vi "GetClickSelection.vi"(1 "Boundaries":cluster{"low":i32, "high":i32}[](array[cluster])=[{"low"=10, "high"=22}, {"low"=30, "high"=42}, {"low"=50, "high"=62}], 2 "Mouse":T1) -> (0 "selection":i32)   [LabVIEW 2012]
uses:
  <vilib>/Utility/miscctls.llb/LVMouseTypeDef.ctl
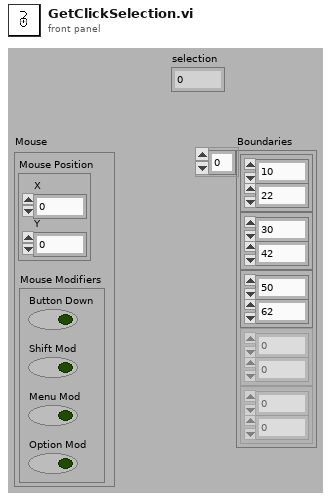
[diagram p1: front panel]
types:
  T1 = typedef "LVMouseTypeDef.ctl" = cluster{"Mouse Position":cluster{"X":i32, "Y":i32}, "Mouse Modifiers":cluster{"Button Down":bool, "Shift Mod":bool, "Menu Mod":bool, "Option Mod":bool}}
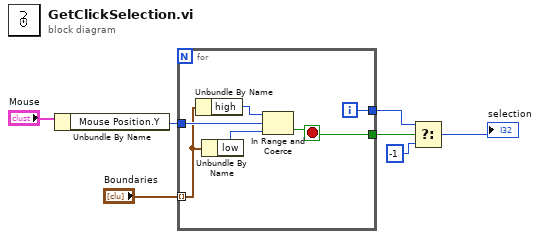
[diagram p0: block diagram]
diagram:
  n1 = Unbundle By Name("Mouse") -> ("Mouse Position.Y"=w5:i32)
  n2 = for {
    tunnel: "Boundaries" -> [w10] mode=indexing
    tunnel: w5 -> [w12]
    tunnel: [w9] -> w3
    tunnel: [w8] -> w4
    i -> [w9]
    stop <- w8 stop-if-true
    n3 = Unbundle By Name(w10) -> ("high"=w13:i32)
    n4 = Unbundle By Name(w10) -> ("low"=w11:i32)
    n5 = In Range and Coerce(upper limit=w13, x=w12, lower limit=w11) -> (In Range?=w8:bool)  [unwired: 1 out]
  }
  n6 = Select(t=w3, s=w4, f=-1) -> (s? t:f=→"selection":i32)
